vi "FTW-Event-Serialize-JSON.vi"(0 "Event Type":string, 5 "Event Data":string, 7 "Source (unwired for call chain, Empty to omit)":string="CallChain", 11 "Error to Log":errorcluster) -> (4 "Serialized Event":string)   [LabVIEW 2013]
panel:
  # "Inputs"
  # "Outputs"
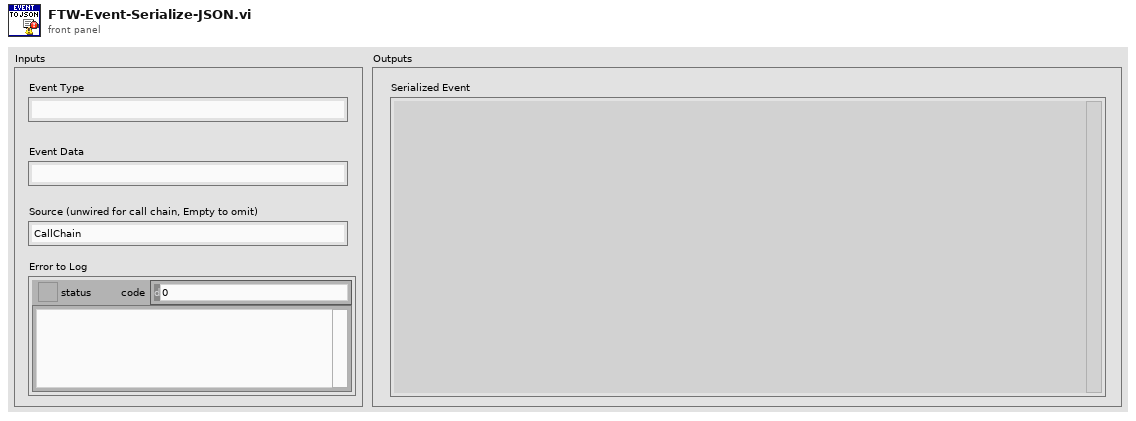
[diagram p1: front panel]
types:
  T1 = typedef "FTW-Event.ctl" = cluster{"Count":i32, "Uptime":dbl, "Timestamp":string, "Source":string, "Type":string, "Data":string, "Error":errorcluster}
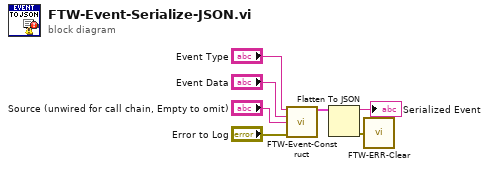
[diagram p0: block diagram]
diagram:
  n1 = call "FTW-Event-Construct.vi"("Event Type"="Event Type", "Event Data"="Event Data", "Source"="Source (unwired for call chain, Empty to omit)", "Error to Log"="Error to Log") -> ("Event"=w3:T1)  [unwired: 11 in]
  n2 = Flatten To JSON(anything=w3) -> (JSON string=→"Serialized Event":string, 11:w1:errorcluster)  [unwired: 2 in]
  n3 = call "FTW-ERR-Clear.vi"("error to snuff"=w1) -> ()  [unwired: 1 out]
